vi "Finish.vi"(4 "error in":errorcluster) -> ()   [LabVIEW 2013]
doc: "This VI is called just before exiting. It is expected to close I/O refnum, save collected data, etc."
uses:
  <vilib>/Rock Robotics/WPI/RobotDrive/WPI_RobotDriveGetSetRefNum.vi
  <vilib>/Rock Robotics/WPI/Joystick/WPI_JoystickGetSetRefNum.vi
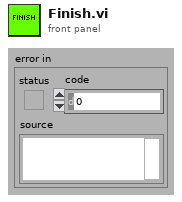
[diagram p1: front panel]
types:
  T1 = typedef "WPI_JoystickDevRef.ctl" = cluster{"Device":T2}
  T2 = typedef "WPI_JoystickDeviceEnum.ctl" = enum16{"USB 1", "USB 2", "USB 3", "USB 4", "Kinect 1", "Kinect 2"}
  T3 = typedef "WPI_CameraDevRef.ctl" = cluster{"Camera Address":string, "CameraStatus":errorcluster, "Acquire Image Notifier":refnum<notifier>}
  T4 = typedef "WPI_RobotDriveDevRef.ctl" = cluster{"DevStatus":errorcluster, "Motors[]":T5[], "Square Inputs":bool, "Max Output":dbl, "Isochronous":bool}
  T5 = typedef "WPI_MotorControlDeviceRef.ctl" = cluster{"DeviceStatus":errorcluster, "Type":enum16{"PWM", "CAN"}, "PWM":cluster{"Digital Module":T6, "PWM Channel":T7, "DeadBand":T8}, "CAN":cluster{"Device Number":u8, "Control Mode":T9, "Semaphore":T10, "Max Vout":dbl}, "Invert":bool, "TransformRef":T11, "InvTransformRef":T11}
  T6 = typedef "FPGA_TypedefDigitalModule.ctl" = enum16{"Digital Module 1", "Digital Module 2"}
  T7 = typedef "FPGA_DIOPWMChannel.ctl" = enum8{"PWM 1", "PWM 2", "PWM 3", "PWM 4", "PWM 5", "PWM 6", "PWM 7", "PWM 8", "PWM 9", "PWM 10", "Invalid"}
  T8 = typedef "WPI_PWMDeadband.ctl" = cluster{"Name":string, "maxPositivePwm":i32, "minPositivePwm":i32, "centerPwm":i32, "maxNegativePwm":i32, "minNegativePwm":i32, "angularRange":u16}
  T9 = typedef "WPI_CANJaguar_ControlMode.ctl" = enum8{"Percent VBus", "Current", "Speed", "Position", "Voltage"}
  T10 = typedef "Semaphore RefNum" = refnum<k1>
  T11 = typedef "WPI_PWMTransform_ConPane.ctl" = refnum<vi>
  T12 = typedef "WPI_EncoderDevRef.ctl" = cluster{"DevStatus":errorcluster, "EncoderIndex":T13, "CounterIndex":T14, "DistancePerCount":dbl, "Decoding Type":T15}
  T13 = typedef "FPGA_EncoderIdx.ctl" = enum8{"Enc 0", "Enc 1", "Enc 2", "Enc 3", "Invalid"}
  T14 = typedef "FPGA_CounterCtrSystemIndex.ctl" = enum8{"Ctr 0", "Ctr 1", "Ctr 2", "Ctr 3", "Ctr 4", "Ctr 5", "Ctr 6", "Ctr 7", "Invalid"}
  T15 = typedef "WPI_EncoderType.ctl" = enum16{"1x", "2x", "4x"}
  T16 = typedef "WPI_SolenoidDevRef.ctl" = cluster{"DevStatus":errorcluster, "Solenoid Module":T17, "Forward Solenoid Channel":T18, "Reverse Solenoid Channel":T18}
  T17 = typedef "FPGA_TypedefSolenoidModule.ctl" = enum16{"Solenoid Module 1", "Solenoid Module 2"}
  T18 = typedef "WPI_SolenoidChannel.ctl" = enum8{"Solenoid 1", "Solenoid 2", "Solenoid 3", "Solenoid 4", "Solenoid 5", "Solenoid 6", "Solenoid 7", "Solenoid 8", "Invalid"}
  T19 = typedef "WPI_DigitalInputDevRef.ctl" = cluster{"DevStatus":errorcluster, "DIO Channel":T20, "Digital Module":T6}
  T20 = typedef "FPGA_DIOChannel.ctl" = enum8{"DIO 1", "DIO 2", "DIO 3", "DIO 4", "DIO 5", "DIO 6", "DIO 7", "DIO 8", "DIO 9", "DIO 10", "DIO 11", "DIO 12", "DIO 13", "DIO 14", "Invalid"}
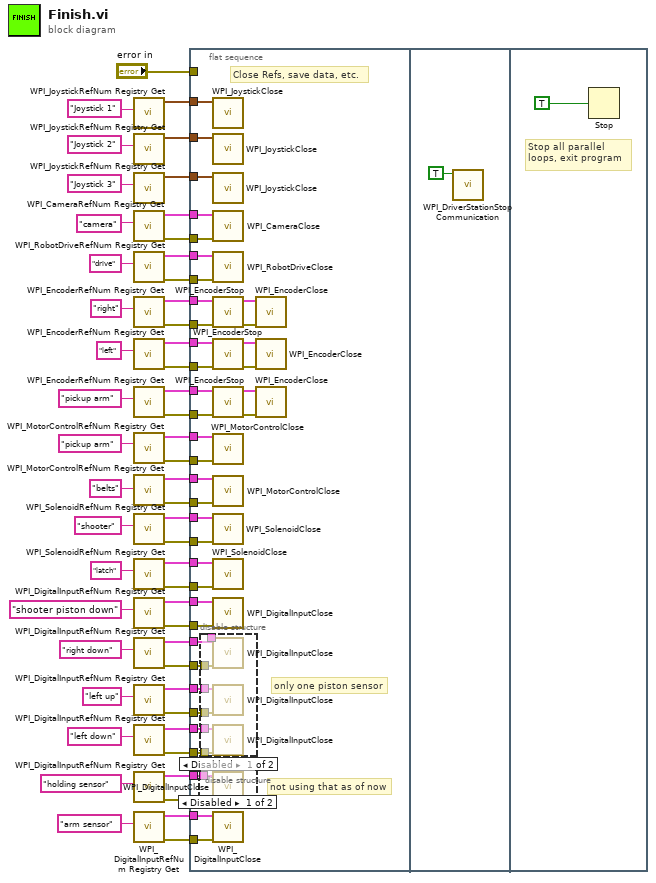
[diagram p0: block diagram]
diagram:
  n1 = call <vilib>:"WPI_JoystickRefNum Registry Get.vi"("refnum name"="Joystick 1") -> ("JoystickDevRef"=w51:T1)  [unwired: 1 in, 9 out]
  n2 = call <vilib>:"WPI_JoystickRefNum Registry Get.vi"("refnum name"="Joystick 2") -> ("JoystickDevRef"=w48:T1)  [unwired: 1 in, 9 out]
  n3 = call <vilib>:"WPI_JoystickRefNum Registry Get.vi"("refnum name"="Joystick 3") -> ("JoystickDevRef"=w45:T1)  [unwired: 1 in, 9 out]
  n4 = call <vilib>:"WPI_CameraRefNum Registry Get.vi"("refnum name"="camera") -> ("error out"=w38:errorcluster, "CameraDevRef"=w50:T3)  [unwired: 1 in, 8 out]
  n5 = call <vilib>:"WPI_RobotDriveRefNum Registry Get.vi"("refnum name"="drive") -> ("error out"=w37:errorcluster, "RobotDriveDevRef"=w43:T4)  [unwired: 9 in]
  n6 = call <vilib>:"WPI_EncoderRefNum Registry Get.vi"("refnum name"="right") -> ("error out"=w36:errorcluster, "EncoderDevRef"=w40:T12)  [unwired: 9 in]
  n7 = call <vilib>:"WPI_EncoderRefNum Registry Get.vi"("refnum name"="left") -> ("error out"=w35:errorcluster, "EncoderDevRef"=w39:T12)  [unwired: 9 in]
  n8 = call <vilib>:"WPI_EncoderRefNum Registry Get.vi"("refnum name"="pickup arm") -> ("error out"=w34:errorcluster, "EncoderDevRef"=w32:T12)  [unwired: 9 in]
  n9 = call <vilib>:"WPI_MotorControlRefNum Registry Get.vi"("refnum name"="pickup arm") -> ("error out"=w28:errorcluster, "MotorControlDevRef"=w29:T5)  [unwired: 9 in]
  n10 = call <vilib>:"WPI_MotorControlRefNum Registry Get.vi"("refnum name"="belts") -> ("error out"=w26:errorcluster, "MotorControlDevRef"=w27:T5)  [unwired: 9 in]
  n11 = call <vilib>:"WPI_SolenoidRefNum Registry Get.vi"("refnum name"="shooter") -> ("error out"=w24:errorcluster, "SolenoidDevRef"=w25:T16)  [unwired: 9 in]
  n12 = call <vilib>:"WPI_SolenoidRefNum Registry Get.vi"("refnum name"="latch") -> ("error out"=w20:errorcluster, "SolenoidDevRef"=w21:T16)  [unwired: 9 in]
  n13 = call <vilib>:"WPI_DigitalInputRefNum Registry Get.vi"("refnum name"="shooter piston down") -> ("error out"=w13:errorcluster, "DigitalInputDevRef"=w14:T19)  [unwired: 9 in]
  n14 = call <vilib>:"WPI_DigitalInputRefNum Registry Get.vi"("refnum name"="right down") -> ("error out"=w11:errorcluster, "DigitalInputDevRef"=w12:T19)  [unwired: 9 in]
  n15 = call <vilib>:"WPI_DigitalInputRefNum Registry Get.vi"("refnum name"="left up") -> ("error out"=w9:errorcluster, "DigitalInputDevRef"=w10:T19)  [unwired: 9 in]
  n16 = call <vilib>:"WPI_DigitalInputRefNum Registry Get.vi"("refnum name"="left down") -> ("error out"=w7:errorcluster, "DigitalInputDevRef"=w8:T19)  [unwired: 9 in]
  n17 = call <vilib>:"WPI_DigitalInputRefNum Registry Get.vi"("refnum name"="holding sensor") -> ("error out"=w4:errorcluster, "DigitalInputDevRef"=w3:T19)  [unwired: 9 in]
  n18 = call <vilib>:"WPI_DigitalInputRefNum Registry Get.vi"("refnum name"="arm sensor") -> ("error out"=w6:errorcluster, "DigitalInputDevRef"=w5:T19)  [unwired: 9 in]
  n19 = flat-sequence {
    tunnel: w51 -> [w91]
    tunnel: w50 -> [w90]
    tunnel: w48 -> [w89]
    tunnel: w45 -> [w88]
    tunnel: w43 -> [w87]
    tunnel: w40 -> [w86]
    tunnel: w39 -> [w79]
    tunnel: w38 -> [w83]
    tunnel: w37 -> [w82]
    tunnel: w36 -> [w81]
    tunnel: w35 -> [w80]
    tunnel: w34 -> [w75]
    tunnel: w32 -> [w74]
    tunnel: w29 -> [w72]
    tunnel: w28 -> [w71]
    tunnel: w27 -> [w69]
    tunnel: w26 -> [w70]
    tunnel: w25 -> [w67]
    tunnel: w24 -> [w68]
    tunnel: w21 -> [w65]
    tunnel: w20 -> [w66]
    tunnel: "error in" -> [_]
    tunnel: w14 -> [w60]
    tunnel: w13 -> [w61]
    tunnel: w12 -> [w59]
    tunnel: w11 -> [w62]
    tunnel: w10 -> [w58]
    tunnel: w9 -> [w63]
    tunnel: w8 -> [w57]
    tunnel: w7 -> [w64]
    tunnel: w3 -> [w55]
    tunnel: w4 -> [w54]
    tunnel: w5 -> [w56]
    tunnel: w6 -> [w53]
    frame #0 {
      # "only one piston sensor"
      # "not using that as of now"
      # "Close Refs, save data, etc."
      n20 = disable-structure shown="Disabled" {
        disable-tunnel: w55 -> [w99 _]
        disable-tunnel: w54 -> [w98 _]
        frame Disabled {
          n21 = call <vilib>:"WPI_DigitalInputClose.vi"("error in (no error)"=w98, "DigitalInputDevRef"=w99) -> ()  [unwired: 9 in, 1 out]
        }
        frame Enabled {
        }
      }
      n22 = disable-structure shown="Disabled" {
        disable-tunnel: w64 -> [w97 _]
        disable-tunnel: w63 -> [w96 _]
        disable-tunnel: w62 -> [w95 _]
        disable-tunnel: w59 -> [w94 _]
        disable-tunnel: w58 -> [w93 _]
        disable-tunnel: w57 -> [w92 _]
        frame Disabled {
          n23 = call <vilib>:"WPI_DigitalInputClose.vi"("error in (no error)"=w95, "DigitalInputDevRef"=w94) -> ()  [unwired: 9 in, 1 out]
          n24 = call <vilib>:"WPI_DigitalInputClose.vi"("error in (no error)"=w96, "DigitalInputDevRef"=w93) -> ()  [unwired: 9 in, 1 out]
          n25 = call <vilib>:"WPI_DigitalInputClose.vi"("error in (no error)"=w97, "DigitalInputDevRef"=w92) -> ()  [unwired: 9 in, 1 out]
        }
        frame Enabled {
        }
      }
      n26 = call <vilib>:"WPI_JoystickClose.vi"("JoystickDevRef"=w91) -> ()  [unwired: 11 out]
      n27 = call <vilib>:"WPI_JoystickClose.vi"("JoystickDevRef"=w89) -> ()  [unwired: 11 out]
      n28 = call <vilib>:"WPI_JoystickClose.vi"("JoystickDevRef"=w88) -> ()  [unwired: 11 out]
      n29 = call <vilib>:"WPI_CameraClose.vi"("error in (no error)"=w83, "CameraDevRef"=w90) -> ()  [unwired: 10 out]
      n30 = call <vilib>:"WPI_RobotDriveClose.vi"("error in (no error)"=w82, "RobotDriveDevRef"=w87) -> ()  [unwired: 9 in, 1 out]
      n31 = call <vilib>:"WPI_EncoderStop.vi"("error in (no error)"=w81, "EncoderDevRef"=w86) -> ("error out"=w85:errorcluster, "EncoderDevRef"=w84:T12)  [unwired: 8 in]
      n32 = call <vilib>:"WPI_EncoderStop.vi"("error in (no error)"=w80, "EncoderDevRef"=w79) -> ("error out"=w77:errorcluster, "EncoderDevRef"=w78:T12)  [unwired: 8 in]
      n33 = call <vilib>:"WPI_EncoderStop.vi"("error in (no error)"=w75, "EncoderDevRef"=w74) -> ("error out"=w76:errorcluster, "EncoderDevRef"=w73:T12)  [unwired: 8 in]
      n34 = call <vilib>:"WPI_MotorControlClose.vi"("error in (no error)"=w71, "MotorControlDevRef"=w72) -> ()  [unwired: 9 in, 1 out]
      n35 = call <vilib>:"WPI_MotorControlClose.vi"("error in (no error)"=w70, "MotorControlDevRef"=w69) -> ()  [unwired: 9 in, 1 out]
      n36 = call <vilib>:"WPI_SolenoidClose.vi"("error in (no error)"=w68, "SolenoidDevRef"=w67) -> ()  [unwired: 9 in, 1 out]
      n37 = call <vilib>:"WPI_SolenoidClose.vi"("error in (no error)"=w66, "SolenoidDevRef"=w65) -> ()  [unwired: 9 in, 1 out]
      n38 = call <vilib>:"WPI_DigitalInputClose.vi"("error in (no error)"=w61, "DigitalInputDevRef"=w60) -> ()  [unwired: 9 in, 1 out]
      n39 = call <vilib>:"WPI_DigitalInputClose.vi"("error in (no error)"=w53, "DigitalInputDevRef"=w56) -> ()  [unwired: 9 in, 1 out]
      n40 = call <vilib>:"WPI_EncoderClose.vi"("error in (no error)"=w85, "EncoderDevRef"=w84) -> ()  [unwired: 9 in, 1 out]
      n41 = call <vilib>:"WPI_EncoderClose.vi"("error in (no error)"=w77, "EncoderDevRef"=w78) -> ()  [unwired: 9 in, 1 out]
      n42 = call <vilib>:"WPI_EncoderClose.vi"("error in (no error)"=w76, "EncoderDevRef"=w73) -> ()  [unwired: 9 in, 1 out]
    }
    frame #1 {
      n43 = call <vilib>:"WPI_DriverStationStop Communication.vi"("StopCommunication"=TRUE) -> ()  [unwired: 10 in, 1 out]
    }
    frame #2 {
      # "Stop all parallel\nloops, exit program"
      n44 = Stop(stop? (T)=TRUE ("Quit")) -> ()
    }
  }
